vi "Find_Cameras.vi"(8 "error in (no error)":errorcluster) -> (0 "error out":errorcluster, 1 "Cam Models":string[](array[string]), 2 "Cam Aliases":string[](array[string]), 3 "Boolean":bool)   [LabVIEW 2023, in "CameraLibrary.lvlib" / "Camera_Controller.lvlib"]
uses:
  Camera_Controller.lvlib
  <vilib>/vision/driver/NI_Vision_Acquisition_Software.lvlib
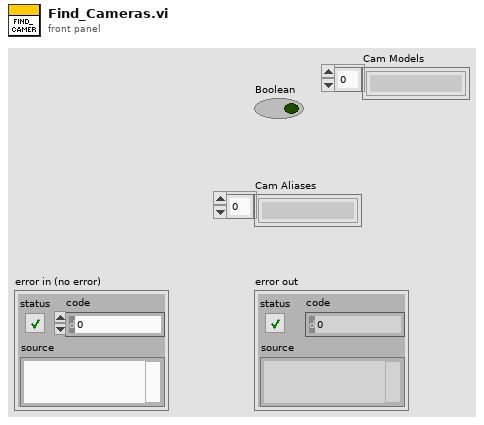
[diagram p1: front panel]
types:
  T1 = cluster{"Type":u32, "Version":u32, "Flags":u32, "SerialNumberHigh":u32, "SerialNumberLow":u32, "BusType":u32, "InterfaceName":string, "VendorName":string, "ModelName":string, "CameraFileName":string, "CameraAttributeURL":string}[]
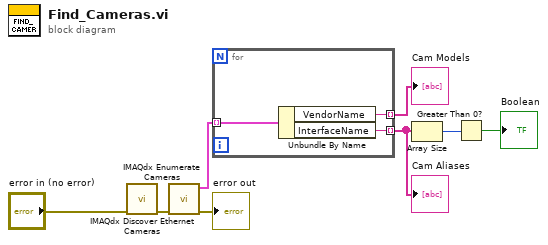
[diagram p0: block diagram]
diagram:
  n1 = call <vilib>:"IMAQdx Discover Ethernet Cameras.vi"("error in"="error in (no error)") -> ("error out"=w2:errorcluster)  [unwired: 10 in]
  n2 = call <vilib>:"IMAQdx Enumerate Cameras.vi"("error in"=w2) -> ("error out"=→"error out":errorcluster, "Camera Information Array"=w3:T1)  [unwired: 9 in]
  n3 = for {
    tunnel: w3 -> [w11] mode=indexing
    tunnel: [w10] -> w7 mode=indexing
    tunnel: [w9] -> w1 mode=indexing
    n4 = Unbundle By Name(w11) -> ("VendorName"=w9:string, "InterfaceName"=w10:string)
  }
  "Cam Aliases" <- w7
  "Cam Models" <- w1
  n5 = Array Size(array=w7) -> (size(s)=w6:i32)
  n6 = Greater Than 0?(x=w6) -> (x > 0?=→"Boolean":bool)
